vi "GEOM_PickFormat.vi"(9 "requested format":string, 10 "default format in":string) -> (0 "detrows":i32, 1 "detcols":i32, 2 "format out":string)   [LabVIEW 2016]
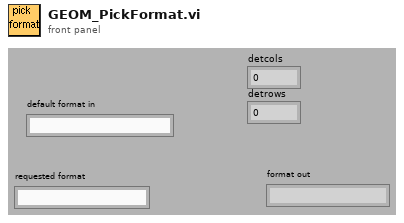
[diagram p1: front panel]
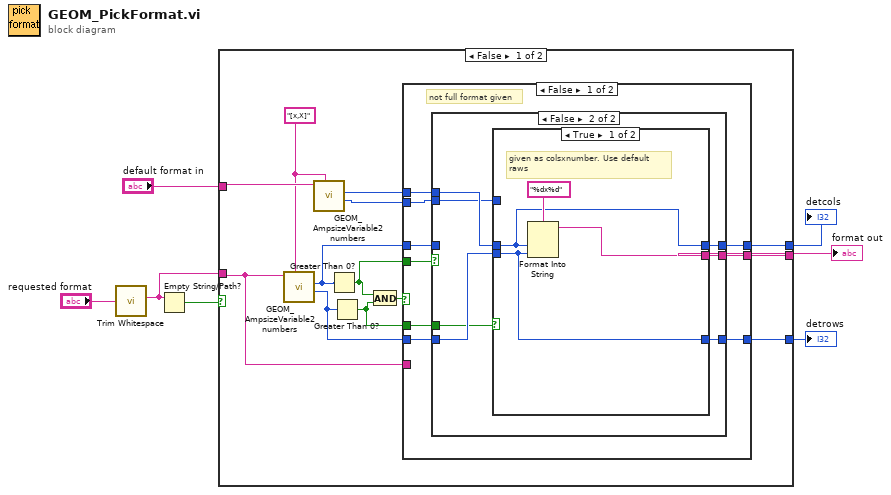
[diagram p0: block diagram]
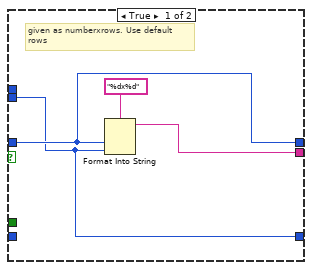
[diagram p2: hidden frame]
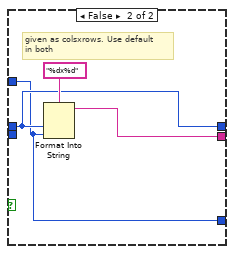
[diagram p3: hidden frame]
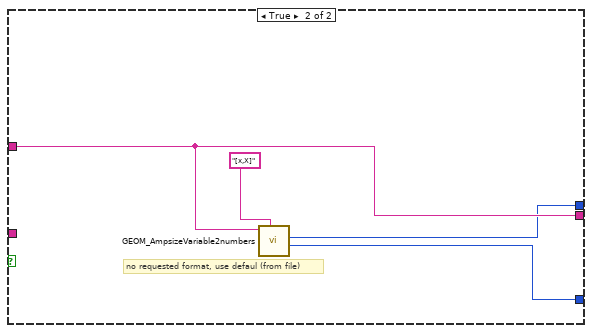
[diagram p5: hidden frame]
diagram:
  n1 = call <vilib>:"Trim Whitespace.vi"("string"="requested format") -> ("trimmed string"=w3:string)  [unwired: 1 in]
  n2 = Empty String/Path?(string/path=w3) -> (empty?=w6:bool)
  n3 = case shown="False" w6 {
    tunnel: "default format in" -> [w15 w54]
    tunnel: [w18 w54] -> w4
    tunnel: w3 -> [w19 _]
    tunnel: [w9 w53] -> w2
    tunnel: [w8 w52] -> w1
    frame False {
      w14 = "[x,X]" ("separator")
      n4 = call "GEOM_AmpsizeVariable2numbers.vi"("separator"=w14, "ampval"=w19) -> ("amprows"=w11:i32, "ampcols"=w16:i32)  [unwired: 2 in, 6 out]
      n5 = call "GEOM_AmpsizeVariable2numbers.vi"("separator"=w14, "ampval"=w15) -> ("amprows"=w12:i32, "ampcols"=w13:i32)  [unwired: 2 in, 6 out]
      n6 = Greater Than 0?(x=w16) -> (x > 0?=w17:bool)
      n7 = Greater Than 0?(x=w11) -> (x > 0?=w10:bool)
      n8 = And(x=w17, y=w10) -> (x .and. y?=w20:bool)
      n9 = case shown="False" w20 {
        tunnel: w19 -> [_ w51]
        tunnel: [w25 w51] -> w18
        tunnel: w17 -> [w29 _]
        tunnel: w16 -> [w28 w50]
        tunnel: w13 -> [w27 _]
        tunnel: w12 -> [w26 _]
        tunnel: w11 -> [w24 w49]
        tunnel: w10 -> [w23 _]
        tunnel: [w22 w50] -> w9
        tunnel: [w21 w49] -> w8
        frame False {
          # "not full format given"
          n10 = case shown="False" w29 {
            tunnel: w28 -> [w31 _]
            tunnel: w27 -> [_ w39]
            tunnel: w26 -> [w30 w36]
            tunnel: [w32 w40] -> w25
            tunnel: w24 -> [_ w38]
            tunnel: w23 -> [_ w37]
            tunnel: [w31 w35] -> w22
            tunnel: [w30 w34] -> w21
            frame True {
              # "given as numberxrows. Use default\nrows"
              n11 = Format Into String(format string="%dx%d", w31, w30) -> (resulting string=w32:string)  [unwired: 2 in, 1 out]
            }
            frame False {
              n12 = case shown="True" w37 {
                tunnel: [w43 w47] -> w40
                tunnel: w39 -> [w42 w46]
                tunnel: w38 -> [w41 _]
                tunnel: w36 -> [_ w45]
                tunnel: [w42 w46] -> w35
                tunnel: [w41 w45] -> w34
                frame True {
                  # "given as colsxnumber. Use default\nraws"
                  n13 = Format Into String(format string="%dx%d", w42, w41) -> (resulting string=w43:string)  [unwired: 2 in, 1 out]
                }
                frame False {
                  # "given as colsxrows. Use default\nin both"
                  n14 = Format Into String(format string="%dx%d", w46, w45) -> (resulting string=w47:string)  [unwired: 2 in, 1 out]
                }
              }
            }
          }
        }
        frame True {
          # "fully format given\n(numberxnumber), use this"
        }
      }
    }
    frame True {
      # "no requested format, use defaul (from file)"
      n15 = call "GEOM_AmpsizeVariable2numbers.vi"("separator"="[x,X]", "ampval"=w54) -> ("amprows"=w52:i32, "ampcols"=w53:i32)  [unwired: 2 in, 6 out]
    }
  }
  "format out" <- w4
  "detcols" <- w2
  "detrows" <- w1
